vi "Conductus Read Heater.vi"(1 "Instrument Address":refnum<visa-resource-name>) -> (0 "Heater Power %":dbl[](array[numeric]) format="%.2f")   [LabVIEW 2024]
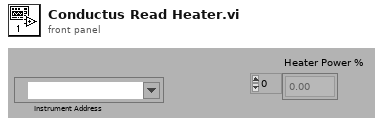
[diagram p1: front panel]
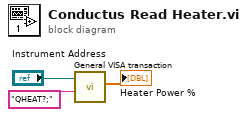
[diagram p0: block diagram]
diagram:
  n1 = call "General VISA transaction.vi"("Command String"="QHEAT?;", "VISA Session"="Instrument Address") -> ("Measurement"=→"Heater Power %":dbl[])  [unwired: 4 in, 5 out]
